vi "显示温度风扇.vi"(7 "Value":variant, 9 "索引":i32, 10 "类别":string, 11 "Tab Control":refnum<vi>) -> ()   [LabVIEW 2015]
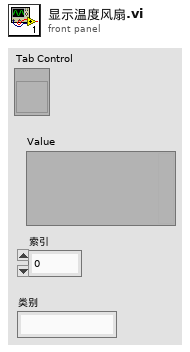
[diagram p1: front panel]
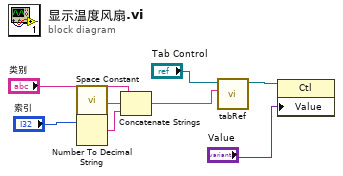
[diagram p0: block diagram]
diagram:
  n1 = call <vilib>:"Space Constant.vi"() -> ("String"=w8:string)
  n2 = Number To Decimal String(number="索引") -> (decimal integer string=w7:string)  [unwired: 1 in]
  n3 = Concatenate Strings("类别", w8, w7) -> (w4:string)
  n4 = call "tabRef.vi"("control name"=w4, "Tab Control"="Tab Control") -> ("control refnum"=w5:refnum<vi>)  [unwired: 8 in, 1 out]
  n5 = property class="Ctl"(reference=w5, "Value"="Value") -> ()  [unwired: 1 in, 2 out]
